vi "add img.vi"(7 "error in (no error)":errorcluster caption="Fehler (Eingang, kein Fehler)", 8 "img.lvclass":refnum<class "img.lvclass">, 10 "Test (Eingang)":refnum<class "Test.lvclass">) -> (0 "error out":errorcluster caption="Fehler (Ausgang)", 3 "Test (Ausgang)":refnum<class "Test.lvclass">)   [LabVIEW 2013, in "DatenKlassen.lvlib" / "Test.lvclass"]
uses:
  Test.lvclass
  Image/img.lvclass
  Test.lvclass/Test.ctl
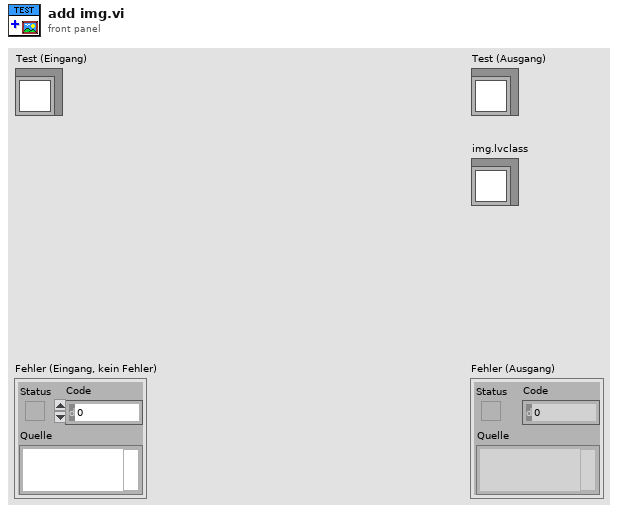
[diagram p1: front panel]
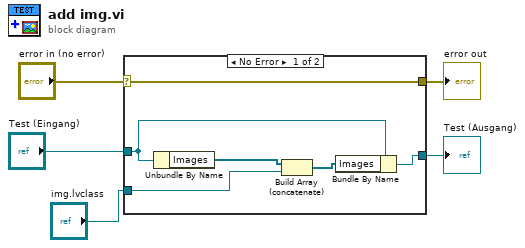
[diagram p0: block diagram]
diagram:
  n1 = case shown="No Error" "error in (no error)" {
    selector: "error in (no error)" -> [w11 w12]
    tunnel: [w11 w12] -> w4
    tunnel: [w9 w13] -> w2
    tunnel: "Test (Eingang)" -> [w8 w13]
    tunnel: "img.lvclass" -> [w6 _]
    frame No Error {
      n2 = Unbundle By Name(w8) -> ("Images"=w10:refnum<class "img.lvclass">[])
      n3 = Build Array (concatenate)(w10, w6) -> (w7:refnum<class "img.lvclass">[])
      n4 = Bundle By Name(cluster=w8, "Images"=w7) -> (w9:refnum<class "Test.lvclass">)
    }
    frame Error {
    }
  }
  "error out" <- w4
  "Test (Ausgang)" <- w2
